vi "ReadTree.vi"(8 "error in":errorcluster, 10 "root":T1, 11 "cRIO repo in":refnum<class "database file.lvclass">) -> (0 "error out":errorcluster, 3 "repository out":refnum<class "NISE_CEF_Repository.lvclass">)   [LabVIEW 2013, in "database file.lvclass"]
uses:
  database file.lvclass
  <vilib>/NI/Configuration Framework/Repository/NISE_CEF_Repository.lvclass
  <vilib>/NI/Configuration Framework/Node/NodeRef.ctl
  <vilib>/NI/Configuration Framework/Node/NISE_CEF_Node.lvclass
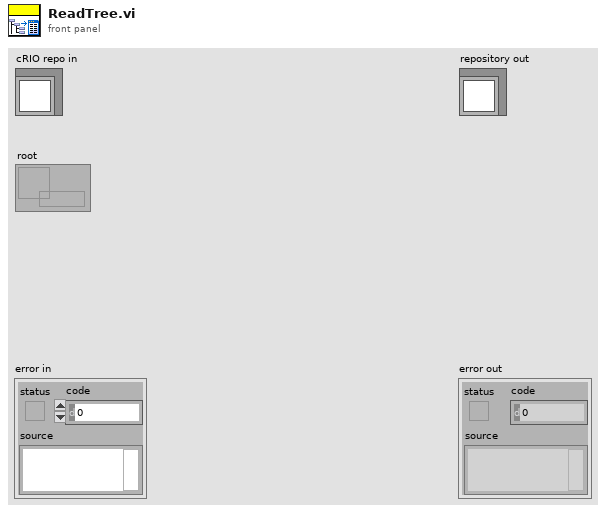
[diagram p1: front panel]
types:
  T1 = typedef "NISE_CEF_Node.lvclass/NodeRef.ctl" = refnum<data-value>
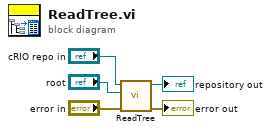
[diagram p0: block diagram]
diagram:
  n1 = call-parent "ReadTree.vi"("error in"="error in", "root"="root", "repository in"="cRIO repo in") -> ("error out"=→"error out":errorcluster, "repository out"=→"repository out":refnum<class "NISE_CEF_Repository.lvclass">)  [unwired: 7 in]
